vi "FGV_HovaCAL_Interface_GetData.vi"(5 "first flags in":T1, 6 "Aktion":T8, 7 "reset index":i32=2, 8 "Limits Cluster in":cluster{"flow":dbl[], "temp":dbl[]}, 9 "actual Values Cluster in":T6 {"Cluster"."PumpModeGeneral-Cluster"."dry mode" items=["wet", "dry"]; "Cluster"."PumpModeGeneral-Cluster"."control mode" items=["static", "pid"]; "Cluster"."PumpMode-Cluster"."concentratio mode" items=["water", "reagent"]; "Cluster"."PumpMode-Cluster"."Reagent" items=["HCl", "HF", "NH3", "HG", "PPM", "ORGANIC"]}, 10 "MFC Flow Cluster in":cluster{"min flow":dbl, "max flow":dbl}[](array[cluster]) {"max flow" format="%.2f"; "min flow" format="%.2f"}, 11 "System Cluster in":T7) -> (0 "Limits Cluster out":cluster{"flow":dbl[], "temp":dbl[]}, 1 "actual Values Cluster out":T6 {"Cluster"."PumpModeGeneral-Cluster"."dry mode" items=["wet", "dry"]; "Cluster"."PumpModeGeneral-Cluster"."control mode" items=["static", "pid"]; "Cluster"."PumpMode-Cluster"."concentratio mode" items=["water", "reagent"]; "Cluster"."PumpMode-Cluster"."Reagent" items=["HCl", "HF", "NH3", "HG", "PPM", "ORGANIC"]}, 2 "MFC Flow Cluster out":cluster{"min flow":dbl, "max flow":dbl}[](array[cluster]), 3 "System Cluster out":T7, 4 "first flags out":T1)   [LabVIEW 2020, in "Linearisierung v2.lvlib" / "Gasteiler.lvlib" / "HovaCAL_Interface.lvlib" / "Kommunikation.lvlib"]
uses:
  Kommunikation.lvlib
  Aktion_FGV_HovaCAL_Interface_GetData.ctl
  Controls/Info Cluster.ctl
  Controls/Pump Dry Mode.ctl
  Controls/Pump Control Mode.ctl
  Controls/Pump Concentration Mode.ctl
  Controls/Reagent.ctl
  Controls/Controls.lvlib
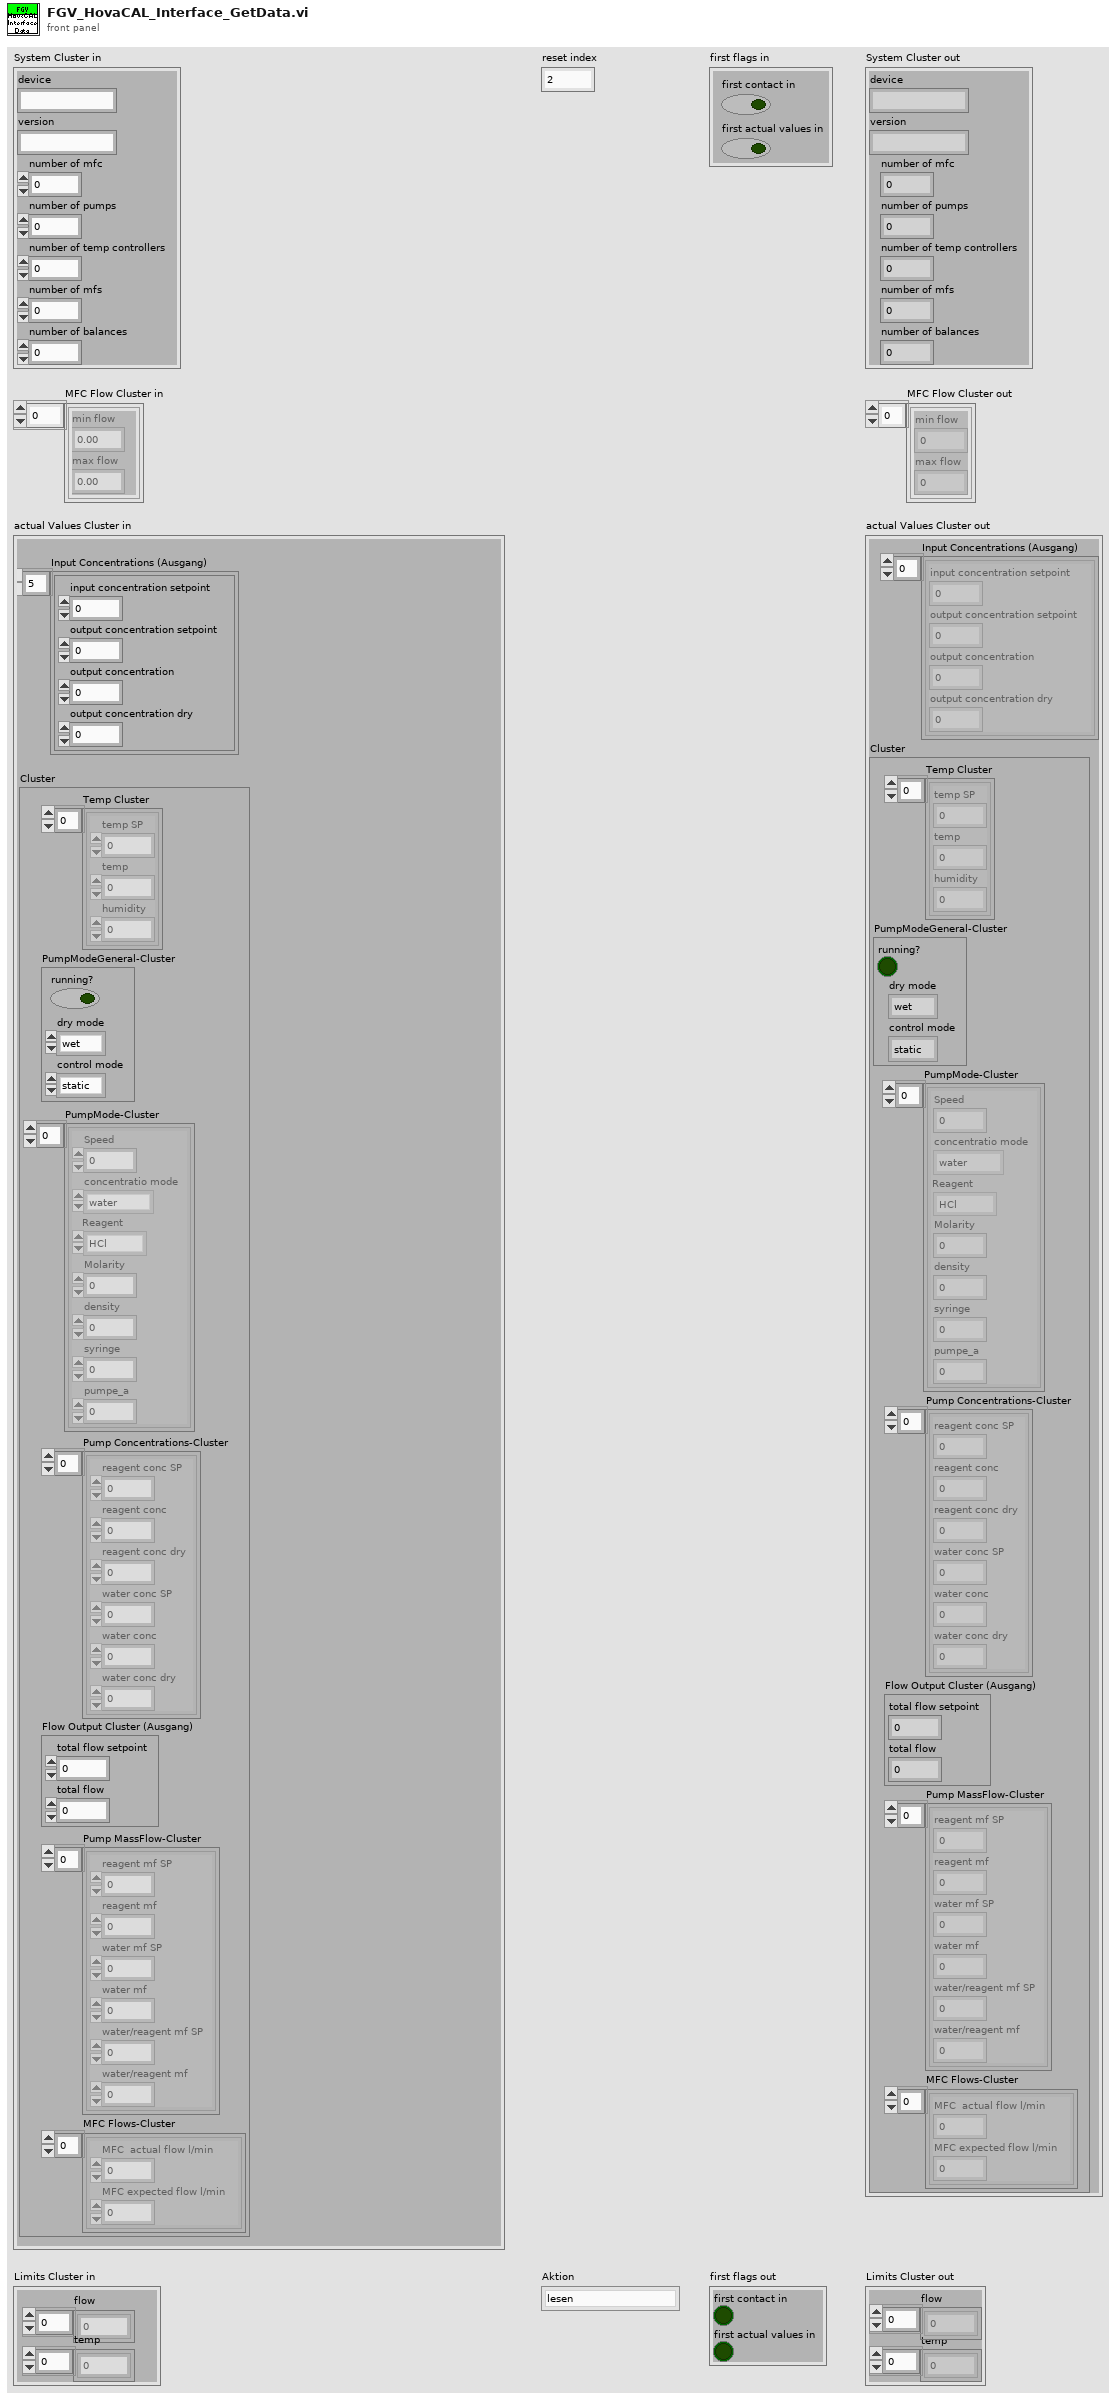
[diagram p1: front panel]
types:
  T1 = cluster{"first contact in":bool, "first actual values in ":bool}
  T2 = typedef "Linearisierung v2.lvlib/Gasteiler.lvlib/HovaCAL_Interface.lvlib/Controls.lvlib/Pump Dry Mode.ctl" = i32
  T3 = typedef "Linearisierung v2.lvlib/Gasteiler.lvlib/HovaCAL_Interface.lvlib/Controls.lvlib/Pump Control Mode.ctl" = u32
  T4 = typedef "Linearisierung v2.lvlib/Gasteiler.lvlib/HovaCAL_Interface.lvlib/Controls.lvlib/Pump Concentration Mode.ctl" = i32
  T5 = typedef "Linearisierung v2.lvlib/Gasteiler.lvlib/HovaCAL_Interface.lvlib/Controls.lvlib/Reagent.ctl" = i32
  T6 = cluster{"Input Concentrations (Ausgang)":cluster{"input concentration setpoint":dbl, "output concentration setpoint":dbl, "output concentration":dbl, "output concentration dry":dbl}[], "Cluster":cluster{"Temp Cluster":cluster{"temp SP":dbl, "temp":dbl, "humidity":dbl}[], "PumpModeGeneral-Cluster":cluster{"running?":bool, "dry mode":T2, "control mode":T3}, "PumpMode-Cluster":cluster{"Speed":dbl, "concentratio mode":T4, "Reagent":T5, "Molarity":dbl, "density":dbl, "syringe":dbl, "pumpe_a":dbl}[], "Pump Concentrations-Cluster":cluster{"reagent conc SP":dbl, "reagent conc":dbl, "reagent conc dry":dbl, "water conc SP":dbl, "water conc":dbl, "water conc dry":dbl}[], "Flow Output Cluster (Ausgang)":cluster{"total flow setpoint":dbl, "total flow":dbl}, "Pump MassFlow-Cluster":cluster{"reagent mf SP":dbl, "reagent mf":dbl, "water mf SP":dbl, "water mf":dbl, "water/reagent mf SP":dbl, "water/reagent mf":dbl}[], "MFC Flows-Cluster":cluster{"MFC  actual flow l/min":dbl, "MFC expected flow l/min":dbl}[]}}
  T7 = typedef "Linearisierung v2.lvlib/Gasteiler.lvlib/HovaCAL_Interface.lvlib/Controls.lvlib/Info Cluster.ctl" = cluster{"device":string, "version":string, "number of mfc":i32, "number of pumps":i32, "number of temp controllers":i32, "number of mfs":i32, "number of balances":i32}
  T8 = typedef "Linearisierung v2.lvlib/Gasteiler.lvlib/HovaCAL_Interface.lvlib/Kommunikation.lvlib/Aktion_FGV_HovaCAL_Interface_GetData.ctl" = enum16{"lesen", "SystemInfo", "MFC Info", "actual Values", "Limits", "first contact", "reset after read"}
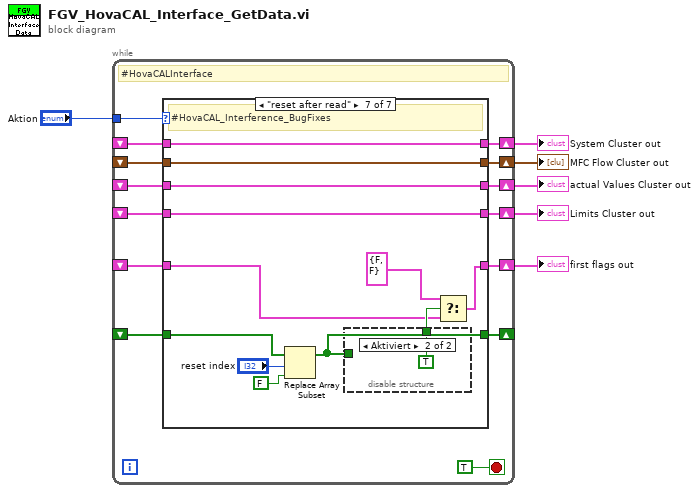
[diagram p0: block diagram]
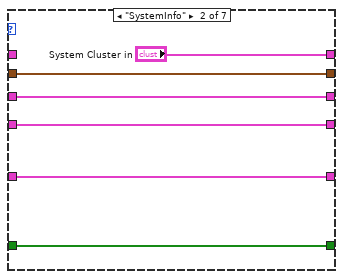
[diagram p3: hidden frame]
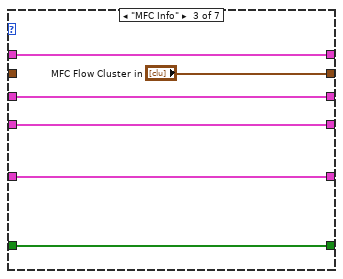
[diagram p4: hidden frame]
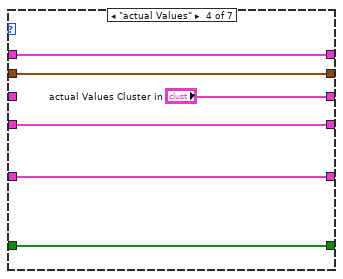
[diagram p5: hidden frame]
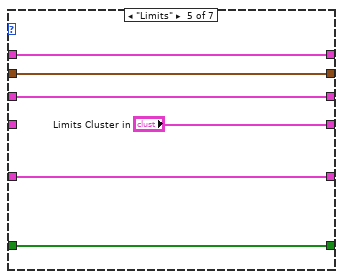
[diagram p6: hidden frame]
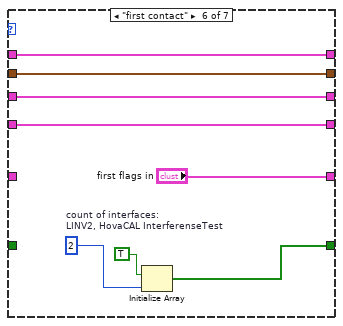
[diagram p7: hidden frame]
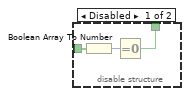
[diagram p8: hidden frame]
diagram:
  n1 = while {
    tunnel: "Aktion" -> [w19]
    shift-right: [w18] -> w5
    shift-left: _ -> [w17]
    shift-right: [w16] -> w4
    shift-left: _ -> [w15]
    shift-right: [w14] -> w3
    shift-left: _ -> [w13]
    shift-right: [w12] -> w2
    shift-left: _ -> [w11]
    shift-right: [w10] -> w1
    shift-left: _ -> [w9]
    shift-right: [w8] -> _
    shift-left: _ -> [w7]
    stop <- TRUE stop-if-true
    # "#HovaCALInterface"
    n2 = case shown="\"reset after read\"" w19 {
      tunnel: [w26 "System Cluster in" w38 w44 w50 w58 w70] -> w18
      tunnel: w17 -> [w26 _ w38 w44 w50 w58 w70]
      tunnel: [w25 w31 "MFC Flow Cluster in" w43 w49 w57 w69] -> w16
      tunnel: w15 -> [w25 w31 _ w43 w49 w57 w69]
      tunnel: [w24 w30 w36 "actual Values Cluster in" w48 w56 w68] -> w14
      tunnel: w13 -> [w24 w30 w36 _ w48 w56 w68]
      tunnel: [w23 w29 w35 w41 "Limits Cluster in" w55 w67] -> w12
      tunnel: w11 -> [w23 w29 w35 w41 _ w55 w67]
      tunnel: [w22 w28 w34 w40 w46 "first flags in" w64] -> w10
      tunnel: w9 -> [w22 w28 w34 w40 w46 _ w63]
      tunnel: [w21 w27 w33 w39 w45 w51 w59] -> w8
      tunnel: w7 -> [w21 w27 w33 w39 w45 _ w62]
      frame "lesen", Default {
      }
      frame "SystemInfo" {
      }
      frame "MFC Info" {
      }
      frame "actual Values" {
      }
      frame "Limits" {
      }
      frame "first contact" {
        w53 = 2  # count of interfaces: LINV2, HovaCAL InterferenseTest
        n3 = Initialize Array(TRUE, w53) -> (w51:bool[])
      }
      frame "reset after read" {
        # "#HovaCAL_Interference_BugFixes"
        n4 = Replace Array Subset(array=w62, new element=FALSE, index="reset index") -> (w59:bool[])
        n5 = disable-structure shown="Aktiviert" {
          disable-tunnel: [w73 TRUE] -> w66
          disable-tunnel: w59 -> [w71 _]
          frame Disabled {
            n6 = Boolean Array To Number(Boolean array=w71) -> (number=w72:u32)
            n7 = Equal To 0?(x=w72) -> (x = 0?=w73:bool)
          }
          frame Enabled {
          }
        }
        n8 = Select(t=T1 {"first contact in"=FALSE, "first actual values in "=FALSE} ("first flags in"), s=w66, f=w63) -> (s? t:f=w64:T1)
      }
    }
  }
  "System Cluster out" <- w5
  "MFC Flow Cluster out" <- w4
  "actual Values Cluster out" <- w3
  "Limits Cluster out" <- w2
  "first flags out" <- w1
